vi "oneDtext2arrayPoly.vi"   [LabVIEW 2017]
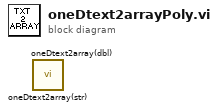
[diagram p0: block diagram]
diagram:
  n1 = call "oneDtext2array(str).vi"() -> ()  [unwired: 12 in]
  n2 = call "oneDtext2array(dbl).vi"() -> ()  [unwired: 11 in, 1 out]
